vi "Reset Headers.vi"(8 "error in (no error)":errorcluster, 9 "NewHeaders":T1[](array[typedef]), 10 "DefaultHeaders":T1[](array[typedef]), 11 "Abstract HTTP Client in":refnum<class "Abstract HTTP Client.lvclass">) -> (0 "error out":errorcluster, 3 "Abstract HTTP Client out":refnum<class "Abstract HTTP Client.lvclass">)   [LabVIEW 2020, in "REST Client.lvlib" / "REST Client.lvclass"]
uses:
  REST Client.lvclass
  REST Client.lvclass/REST Client.ctl
  <vilib>/VIPM Community/HTTP Client Plugin - Base/Classes/Abstract HTTP Client/Abstract HTTP Client.lvclass
  <vilib>/NI/Advanced HTTP Client/Header--Combo Box.ctl
  <vilib>/NI/Advanced HTTP Client/Session.lvclass
  HTTP Header.ctl
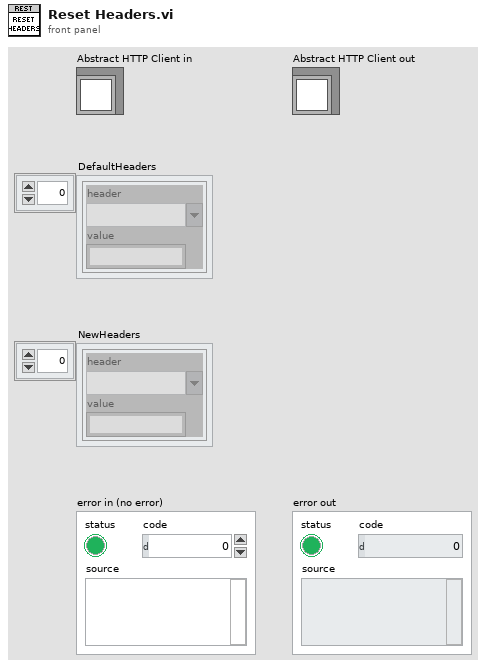
[diagram p1: front panel]
types:
  T1 = typedef "REST Client.lvlib/REST Client.lvclass/HTTP Header.ctl" = cluster{"header":T2, "value":string}
  T2 = typedef "lib_NI_Advanced HTTP Client.lvlib/Session.lvclass/Header--Combo Box.ctl" = string
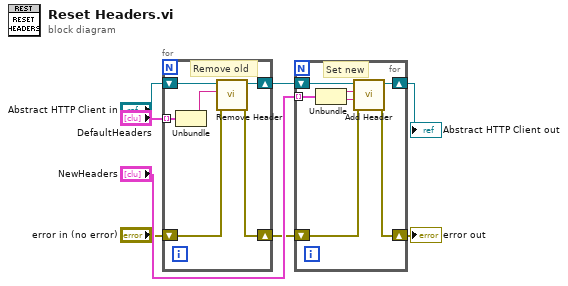
[diagram p0: block diagram]
diagram:
  n1 = for {
    shift-right: [w10] -> w7
    shift-left: "error in (no error)" -> [w11]
    shift-right: [w9] -> w4
    shift-left: "Abstract HTTP Client in" -> [w12]
    tunnel: "DefaultHeaders" -> [w14] mode=indexing
    # "Remove old"
    n2 = Unbundle(w14) -> ("header"=w13:T2)  [unwired: 1 out]
    n3 = call-dynamic "Remove Header.vi"("error in (no error)"=w11, "header"=w13, "HTTP Client Abstract in"=w12) -> ("error out"=w10:errorcluster, "HTTP Client Abstract out"=w9:refnum<class "Abstract HTTP Client.lvclass">)  [unwired: 7 in]
  }
  n4 = for {
    shift-right: [w15] -> w6
    shift-left: w7 -> [w16]
    shift-right: [w19] -> w5
    shift-left: w4 -> [w20]
    tunnel: "NewHeaders" -> [w21] mode=indexing
    # "Set new"
    n5 = Unbundle(w21) -> ("header"=w18:T2, "value"=w17:string)
    n6 = call-dynamic "Add Header.vi"("error in (no error)"=w16, "value"=w17, "header"=w18, "HTTP Client Abstract in"=w20) -> ("error out"=w15:errorcluster, "HTTP Client Abstract out"=w19:refnum<class "Abstract HTTP Client.lvclass">)  [unwired: 6 in]
  }
  "error out" <- w6
  "Abstract HTTP Client out" <- w5
